vi "Find_Rows_To_Average.vi"(2 "Averaging Period":dbl[](array[numeric]) format="%.2f", 3 "Approx Scan Period":dbl=7.0 format="%.2f") -> (0 "Remove top Row":bool, 1 "Index":i32)   [LabVIEW 2010]
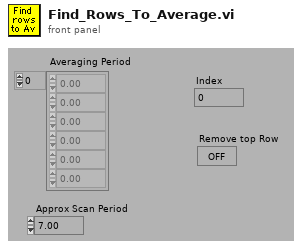
[diagram p1: front panel]
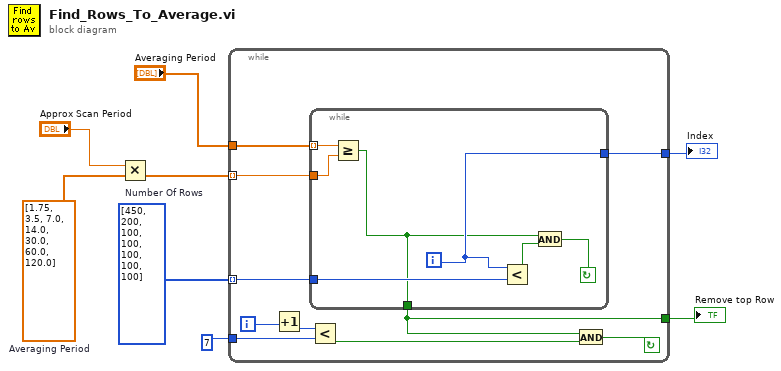
[diagram p0: block diagram]
diagram:
  w7 = i32[] [450, 200, 100, 100, 100, 100, 100]  # Number Of Rows
  w3 = dbl[] [1.75, 3.5, 7.0, 14.0, 30.0, 60.0, 120.0]  # Averaging Period
  n1 = Multiply(x="Approx Scan Period", y=w3) -> (x*y=w1:dbl[])
  n2 = while {
    tunnel: [w9] -> w4
    tunnel: [w10] -> w5
    tunnel: 7 -> [w13]
    tunnel: w7 -> [w16] mode=indexing
    tunnel: w1 -> [w17] mode=indexing
    tunnel: "Averaging Period" -> [w18]
    i -> [w15]
    stop <- w11 continue-if-true
    n3 = Increment(x=w15) -> (x+1=w14:i32)
    n4 = while {
      tunnel: [w19] -> w9
      tunnel: w16 -> [w22]
      tunnel: [w23] -> w10
      tunnel: w17 -> [w24]
      tunnel: w18 -> [w25] mode=indexing
      i -> [w23]
      stop <- w20 continue-if-true
      n5 = Greater Or Equal?(x=w25, y=w24) -> (x >= y?=w19:bool)
      n6 = Less?(x=w23, y=w22) -> (x < y?=w21:bool)
      n7 = And(x=w19, y=w21) -> (x .and. y?=w20:bool)
    }
    n8 = Less?(x=w14, y=w13) -> (x < y?=w12:bool)
    n9 = And(x=w9, y=w12) -> (x .and. y?=w11:bool)
  }
  "Index" <- w5
  "Remove top Row" <- w4
